vi "Main RT.vi"() -> ()   [LabVIEW 2019]
uses:
  <vilib>/Memosfet/myRIO-Neopixel/RT/Display Utilities/Public/Controls/2D Dimensions.ctl
  <vilib>/Memosfet/myRIO-Neopixel/RT/Graph/Graph.lvclass
  C:/Program Files (x86)/National Instruments/LabVIEW 2019/vi.lib/Memosfet/myRIO-Neopixel/RT/Display Element/Display Element.lvclass
  <vilib>/Memosfet/myRIO-Neopixel/RT/Graph/Public/Controls/Fill To.ctl
  <vilib>/Memosfet/myRIO-Neopixel/RT/Display/Public/Controls/RGB Gains.ctl
  <vilib>/FPGAPlugInAG/myRIO-1900/niLvFpga_Open_myRIO-1900.vi
  <vilib>/rvi/interface/common/dynamic/niFpgaDynamicAddResources.vi
  <vilib>/FPGAPlugInAG/Dynamic/niLvFpga_Reset_Dynamic.vi
  <vilib>/Utility/error.llb/Error Cluster From Error Code.vi
  <vilib>/rvi/errors/niLvFpgaAdjustHostInterfaceError.vi
  <vilib>/rvi/Analysis/host/Private/Sample Rate To Loop Time (ticks).vi
  <vilib>/FPGAPlugInAG/Dynamic/niLvFpga_Close_Dynamic.vi
  <vilib>/rvi/interface/nirviOpenFPGA/nirviOpenFPGA.xnode
  Bitfiles/mydashboard_FPGATarget_MainFPGA1_sclqAr1bu20.lvbitx
  <vilib>/rvi/interface/nirviMethod/nirviMethod.xnode
  <vilib>/rvi/interface/nirviReadWriteControl/nirviReadWriteControl.xnode
  <vilib>/rvi/interface/nirviCloseFPGA/nirviCloseFPGA.xnode
  <vilib>/Memosfet/myRIO-Neopixel/RT/Display/Display.lvclass
  <vilib>/rvi/Analysis/host/Public/NI_FpgaMspHost.lvlib
  <vilib>/FPGAPlugInAG/Dynamic/niLvFpga_ReadFifo_Dynamic.vi
  <vilib>/rvi/errors/niLvFpgaMergeErrorWithErrorCode.vi
  <vilib>/Memosfet/myRIO-Neopixel/RT/Display Utilities/Display Utilities.lvlib
  <vilib>/FPGAPlugInAG/Dynamic/niLvFpga_WriteFifo_Dynamic.vi
  NiFpgaLv.dll
  <vilib>/rvi/interface/Simulation/niFpgaSimulationCallBeginRW.vi
panel:
  out "Error Out":errorcluster
  in  "FPS":u32(slide) scale=0.0..100.0
  in  "Gain":sgl(slide)=0.45627376 scale=0.0..1.0
  in  "Stop":bool
  out "Invalid Sample Rate":bool
  out "FFT Spectrum":waveform(dbl)(graph)={"t0"=timestamp(0 s since 1904-01-01), "dt"=312.5, "Y"=[0.02503204345703125, 0.00043494240764585035, 0.00022243316249257283, 0.00013519321553550227, 0.0005238233610159873, 0.00027038643107100453, 0.0002213839436118608, 0.00015448346505215905, 0.0002424659512645066, 0.0001729703376579992, 0.0001862572573201554, 0.00010843406985131756, 0.0003281526667420436, 0.00022243316249257283, 4.315837287515549e-05, 5.394796609394436e-05, 0.00010789593218788873, 0.00010789593218788873, 7.780486318348366e-05, 3.890243159174183e-05, 9.281559036709931e-05, 1.0789593218788873e-05, 8.897326499702913e-05, 0.00010626516935107513, 2.1579186437577746e-05, 8.897326499702913e-05, 4.825252777356536e-05, 8.897326499702913e-05, 1.0789593218788873e-05, 3.051757812500001e-05, 6.823937919616058e-05, 4.825252777356536e-05]}
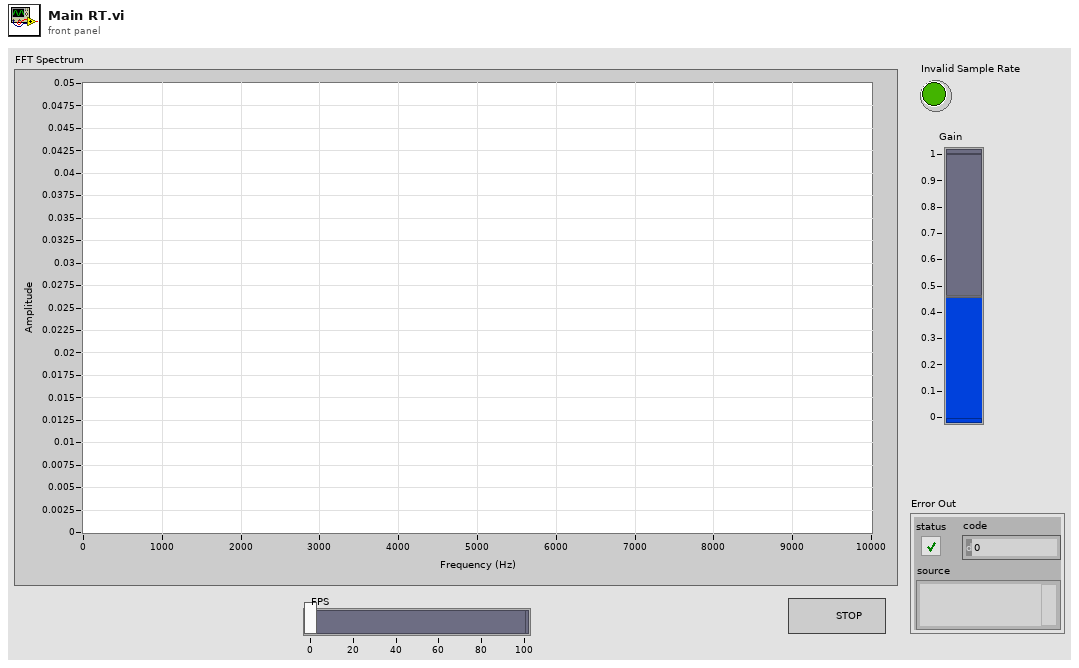
[diagram p1: front panel]
types:
  T1 = typedef "Graph.lvclass/Fill To.ctl" = enum16{"None", "Inf", "-Inf"}
  T2 = typedef "Display Utilities.lvlib/2D Dimensions.ctl" = cluster{"Width":i32, "Height":i32}
  T3 = typedef "Display.lvclass/RGB Gains.ctl" = cluster{"Red":sgl, "Green":sgl, "Blue":sgl}
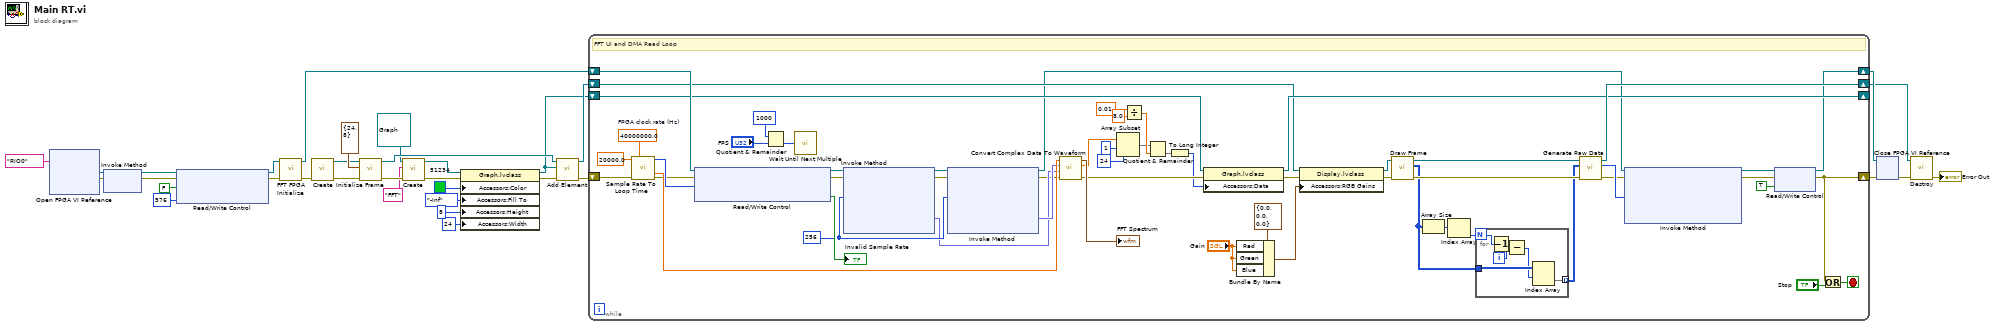
[diagram p0: block diagram]
diagram:
  n1 = xnode "Open FPGA VI Reference"("resource name"=tag "RIO0") -> ("FPGA VI Reference Out"=w29:refnum<k20>, "error out"=w30:errorcluster)  [unwired: 1 in]
  n2 = xnode "Invoke Method"("FPGA VI Reference In"=w29, "error in"=w30) -> ("FPGA VI Reference Out"=w6:refnum<k20>, "error out"=w5:errorcluster)
  n3 = xnode "Read/Write Control"("FPGA VI Reference In"=w6, "error in"=w5, "Update"=FALSE, "Number Of Elements"=576) -> ("FPGA VI Reference Out"=w2:refnum<k20>, "error out"=w3:errorcluster)
  n4 = call "FFT FPGA Initialize.vi"("error in (no error)"=w3, "Refnum in"=w2) -> ("error out"=w20:errorcluster, "Refnum out"=w31:refnum<k20>)  [unwired: 8 in]
  n5 = call <vilib>:"Create.vi"("Error In"=w20) -> ("Error Out"=w25:errorcluster, "Screen Out"=w26:refnum<class "Display.lvclass">)  [unwired: 9 in]
  n6 = call <vilib>:"Initialize Frame.vi"("Error In"=w25, "Size"=T2 {"Width"=24, "Height"=8}, "Display In"=w26) -> ("Error Out"=w24:errorcluster, "Display Out"=w23:refnum<class "Display.lvclass">)  [unwired: 7 in]
  n7 = call-dynamic <vilib>:"Create.vi"("Error In"=w24, "Tag"="FFT", "Graph In"=refnum<class "Graph.lvclass"> refnum) -> ("Error Out"=w14:errorcluster, "Graph Out"=w15:refnum<class "Graph.lvclass">)  [unwired: 7 in]
  n8 = property class="Graph.lvclass"(reference=w15, error in=w14, "Accessors:Color"=u32 51234 ("Color"), "Accessors:Fill To"=Fill_To."-Inf" ("Fill To"), "Accessors:Height"=u32 8 ("Height"), "Accessors:Width"=u32 24 ("Width")) -> (reference out=w8:refnum<class "Graph.lvclass">, error out=w13:errorcluster)
  n9 = call <vilib>:"Add Element.vi"("Error In"=w13, "New Element"=w8, "Display In"=w23) -> ("Error Out"=w19:errorcluster, "Display Out"=w18:refnum<class "Display.lvclass">)  [unwired: 7 in]
  n10 = while {
    shift-right: [w40] -> w33
    shift-left: w31 -> [w79]
    shift-right: [w39] -> w32
    shift-left: w19 -> [w80]
    shift-right: [w70] -> w17
    shift-left: w18 -> [w56]
    shift-right: [w63] -> _
    shift-left: w8 -> [w64]
    stop <- w87 stop-if-true
    w83 = u32 256 ("Number of Elements")
    w78 = 40000000.0  # FPGA clock rate (Hz)
    # "FFT UI and DMA Read Loop"
    n11 = call-poly <vilib>:"Sample Rate To Loop Time.vi"("sample rate (S/s)"=20000.0 ("Sample rate (S/s)"), "FPGA clock rate (Hz)"=w78, "error in (no error)"=w80) -> ("count (ticks/S)"=w77:u32, "actual sample rate (S/s)"=w76:dbl, "error out"=w72:errorcluster)  [unwired: 10 in]
    n12 = xnode "Read/Write Control"("FPGA VI Reference In"=w79, "error in"=w72, "Requested Sample Period (ticks)"=w77) -> ("FPGA VI Reference Out"=w86:refnum<k20>, "error out"=w81:errorcluster, "Invalid Period"=→"Invalid Sample Rate":bool)
    n13 = Quotient & Remainder(x=u32 1000 ("y"), y="FPS") -> (floor(x/y)=w48:u32)  [unwired: 1 out]
    n14 = call "Wait Until Next Multiple"("Count(mSec)"=w48) -> ()  [unwired: 1 out]
    n15 = xnode "Invoke Method"("FPGA VI Reference In"=w86, "error in"=w81, "Number of Elements"=w83) -> ("FPGA VI Reference Out"=w89:refnum<k20>, "error out"=w82:errorcluster, "Data"=w74:fxp<+/-,25,14>[])  [unwired: 1 in, 1 out]
    n16 = xnode "Invoke Method"("FPGA VI Reference In"=w89, "error in"=w82, "Number of Elements"=w83) -> ("FPGA VI Reference Out"=w44:refnum<k20>, "error out"=w73:errorcluster, "Data"=w75:fxp<+/-,25,14>[])  [unwired: 1 in, 1 out]
    n17 = call "Convert Complex Data To Waveform.vi"("error in"=w73, "Real Data"=w74, "Imaginary Data"=w75, "Sample Rate (S/s)"=w76) -> ("error out"=w68:errorcluster, "spectrum out"=w67:dbl[], "Waveform"=→"FFT Spectrum":waveform(dbl))  [unwired: 5 in]
    n18 = Array Subset(array=w67, index=1, length=24) -> (w59:dbl[])
    n19 = Divide(x=0.01, y=8.0) -> (x/y=w60:dbl)
    n20 = Quotient & Remainder(x=w59, y=w60) -> (floor(x/y)=w58:dbl[])  [unwired: 1 out]
    n21 = To Long Integer(number=w58) -> (32bit integer=w57:i32[])
    n22 = property class="Graph.lvclass"(reference=w64, error in=w68, "Accessors:Data"=w57) -> (reference out=w63:refnum<class "Graph.lvclass">, error out=w55:errorcluster)
    n23 = Bundle By Name(cluster=T3 {"Red"=0.0, "Green"=0.0, "Blue"=0.0} ("RGB Gains"), "Red"="Gain", "Green"="Gain", "Blue"="Gain") -> (w50:T3)
    n24 = property class="Display.lvclass"(reference=w56, error in=w55, "Accessors:RGB Gains"=w50) -> (reference out=w54:refnum<class "Display.lvclass">, error out=w53:errorcluster)
    n25 = call <vilib>:"Draw Frame.vi"("Error In"=w53, "Display In"=w54) -> ("Error Out"=w45:errorcluster, "Frame"=w35:u32[][], "Display Out"=w46:refnum<class "Display.lvclass">)  [unwired: 7 in]
    n26 = Array Size(array=w35) -> (size(s)=w37:i32[])
    n27 = Index Array(array=w37) -> (element=w36:i32)  [unwired: 1 in]
    n28 = for {
      N: w36 -> [w92]
      tunnel: w35 -> [w94]
      tunnel: [w90] -> w34 mode=indexing
      i -> [w95]
      n29 = Decrement(x=w92) -> (x-1=w91:i32)
      n30 = Subtract(x=w91, y=w95) -> (x-y=w93:i32)
      n31 = Index Array(array=w94, index (row)=w93) -> (element=w90:u32[])  [unwired: 1 in]
    }
    n32 = call <vilib>:"Generate Raw Data.vi"("Error In"=w45, "Matrix"=w34, "Display In"=w46) -> ("Error Out"=w43:errorcluster, "Raw Data"=w69:u8[], "Display Out"=w70:refnum<class "Display.lvclass">)  [unwired: 6 in]
    n33 = xnode "Invoke Method"("FPGA VI Reference In"=w44, "error in"=w43, "Data"=w69) -> ("FPGA VI Reference Out"=w41:refnum<k20>, "error out"=w42:errorcluster)  [unwired: 1 in, 1 out]
    n34 = xnode "Read/Write Control"("FPGA VI Reference In"=w41, "error in"=w42, "Update"=TRUE) -> ("FPGA VI Reference Out"=w40:refnum<k20>, "error out"=w39:errorcluster)
    n35 = Or(x=w39, y="Stop") -> (x .or. y?=w87:bool)
  }
  n36 = xnode "Close FPGA VI Reference"("FPGA VI Reference In"=w33, "error in"=w32) -> ("error out"=w16:errorcluster)
  n37 = call <vilib>:"Destroy.vi"("Error In"=w16, "Display In"=w17) -> ("Error Out"=→"Error Out":errorcluster)  [unwired: 9 in]
